vi "Write Measurement Values.vi"(0 "Selected Part Name":string="1891", 2 "RC JSON variant in":variant, 5 "Input Data Cluster":T1, 7 "Input File Paths Cluster":T5={"JSON Default filepath in"=path "F:/User Interface Testbench/Configuration file/Zengage System JSON UI.json", "JSON RackController\n(Override) filepath in"=path "F:/User Interface Testbench/Configuration file/Rack Controller Override JSON UI.json", "JSON AlgoParameters\n(Override) filepath in"=path "F:/User Interface Testbench/Configuration file/Algorithm Override JSON.json"}, 9 "Measurements Cluster":T4={"Measurement Values"=[["L", "AET", "16", "2", "10", "2", "10", "1", "0"], ["W", "AET", "2.5", "-10", "100", "-10", "100", "1", "0"], ["I1", "Length", "9.5", "-10", "100", "-10", "100", "1", "0"], ["U", "Coord", "2.3", "2", "20", "-10", "100", "1", "0"]], "Enabled Disable Array"=[]}, 11 "error in":errorcluster, 12 "User interface enqueuer":refnum<class "Message Enqueuer.lvclass">, 13 "Algo JSON variant in":variant) -> (4 "RC JSON variant out":variant, 6 "Algo JSON variant out":variant, 15 "error out":errorcluster)   [LabVIEW 2019, in "ZenGage v3.0 UI.lvclass"]
uses:
  ZenGage v3.0 UI.lvclass
  User Interface Messages/User Interface messages/Display Popup Msg/DisplayPopup_UI.lvclass
  Common/Controls/Pop-up Input.ctl
  <vilib>/ActorFramework/Message Enqueuer/Message Enqueuer.lvclass
  Type Definitions/Edit tolerance settings/Rack Selection.ctl
  <vilib>/Utility/miscctls.llb/LVPoint32TypeDef.ctl
  Type Definitions/Edit tolerance settings/Edit Tolerance Input.ctl
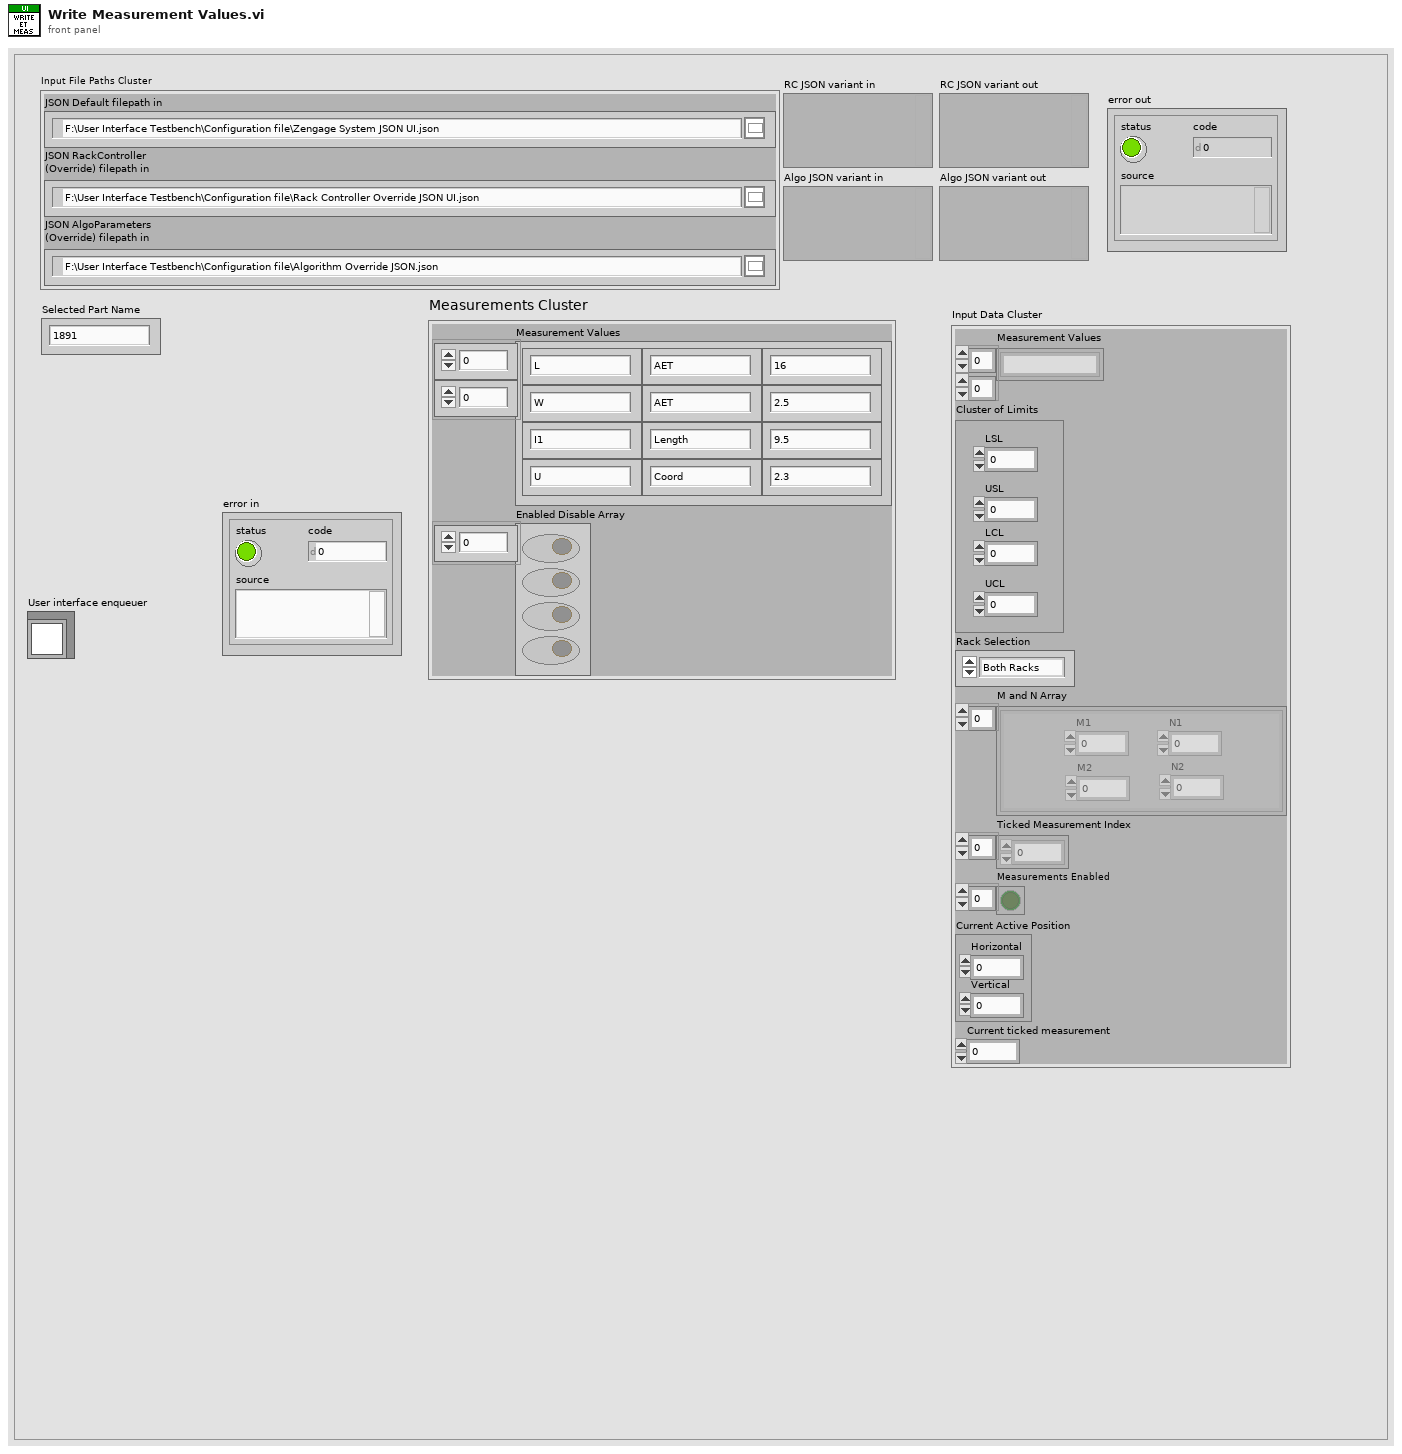
[diagram p1: front panel]
types:
  T1 = typedef "ZenGage v3.0 UI.lvclass/Edit Tolerance Input.ctl" = cluster{"Measurement Values":string[][], "Cluster of Limits":cluster{"LSL":dbl, "USL":dbl, "LCL":dbl, "UCL":dbl}, "Rack Selection":T2, "M and N Array":cluster{"M1":u64, "M2":u64, "N1":u64, "N2":u64}[], "Ticked Measurement Index":u32[], "Measurements Enabled":bool[], "Current Active Position":T3, "Current ticked measurement":dbl}
  T2 = typedef "ZenGage v3.0 UI.lvclass/Rack Selection.ctl" = enum16{"Both Racks", "Rack 2", "Rack 1"}
  T3 = typedef "LVPoint32TypeDef.ctl" = cluster{"Horizontal":i32, "Vertical":i32}
  T4 = cluster{"Measurement Values":string[][], "Enabled Disable Array":bool[]}
  T5 = cluster{"JSON Default filepath in":path, "JSON RackController\n(Override) filepath in":path, "JSON AlgoParameters\n(Override) filepath in":path}
  T6 = typedef "Pop-up Input.ctl" = cluster{"Pop-up Type":enum16{"Open Logo Display", "Close Logo Display", "Open Loading Bar", "Close Loading Bar", "Open Alert Display", "Close Alert Display", "One button dialog box", "Two button dialog box", "User Authentication"}, "Title":string, "Message":string, "Button 1 Text":string, "Button 2 Text":string, "Show Close? T/F":bool, "Title Blink? T/F":bool, "Title Blink Colour":u32}
  T7 = cluster{"Tolerance Limits":dbl[][], "Measurement Enable":bool[], "Bias Correction":dbl[], "Linearity Correction":dbl[], "Measurement names":string[]}
  T8 = cluster{"M1":u64, "M2":u64, "N1":u64, "N2":u64}[]
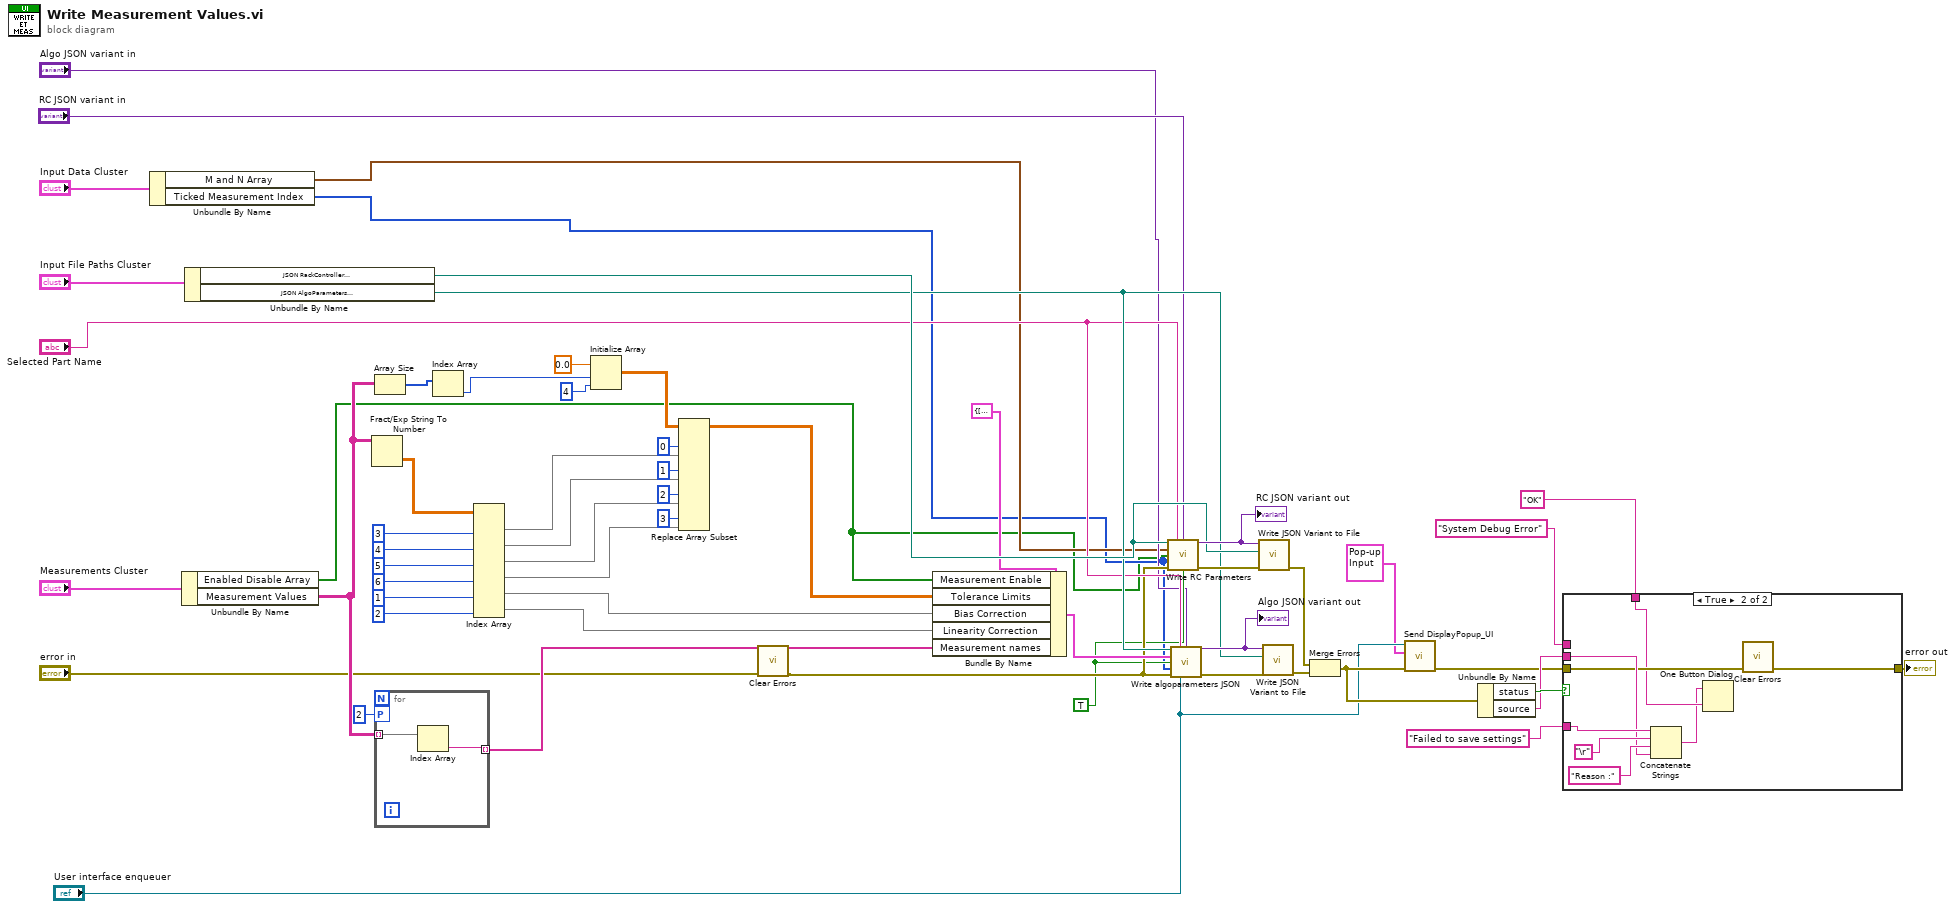
[diagram p0: block diagram]
diagram:
  w12 = TRUE
  n1 = Unbundle By Name("Input Data Cluster") -> ("M and N Array"=w5:T8, "Ticked Measurement Index"=w4:u32[])
  n2 = Unbundle By Name("Measurements Cluster") -> ("Enabled Disable Array"=w1:bool[], "Measurement Values"=w16:string[][])
  n3 = Unbundle By Name("Input File Paths Cluster") -> ("JSON RackController\n(Override) filepath in"=w44:path, "JSON AlgoParameters\n(Override) filepath in"=w43:path)
  n4 = Fract/Exp String To Number(string=w16) -> (number=w54:dbl[][])  [unwired: 3 in, 1 out]
  n5 = Array Size(array=w16) -> (size(s)=w31:i32[])
  n6 = for {
    tunnel: w16 -> [w60] mode=indexing
    tunnel: [w59] -> w15 mode=indexing
    workers-P: 2 -> [_]
    n7 = Index Array(array=w60) -> (element=w59:string)  [unwired: 1 in]
  }
  n8 = Index Array(array=w31) -> (element=w30:i32)  [unwired: 1 in]
  n9 = Index Array(array=w54, index (col) #1=3 ("index (row)"), index (col) #2=4 ("index (row)"), index (col) #3=5 ("index (row)"), index (col) #4=6 ("index (row)"), index (col) #5=1 ("index (row)"), index (col) #6=2 ("index (row)")) -> (element #1=w53:dbl[], element #2=w52:dbl[], element #3=w51:dbl[], element #4=w50:dbl[], element #5=w40:dbl[], element #6=w39:dbl[])  [unwired: 6 in]
  n10 = Initialize Array(0.0, w30, 4 ("dimension size")) -> (w55:dbl[][])
  n11 = Replace Array Subset(array=w55, new element #1=w53, index (col) #1=0 ("disabled index (col)"), new element #2=w52, index (col) #2=1 ("index (col)"), new element #3=w51, index (col) #3=2 ("index (col)"), new element #4=w50, index (col) #4=3 ("index (col)")) -> (w36:dbl[][])  [unwired: 4 in]
  n12 = call <vilib>:"Clear Errors.vi"("error in (no error)"="error in") -> ("error out"=w13:errorcluster)  [unwired: 5 in, 1 out]
  n13 = Bundle By Name(cluster=T7 {"Tolerance Limits"=[[3.9, 4.3, 3.9, 4.3], [15.2, 15.8, 15.2, 15.8], [15.2, 15.8, 15.2, 15.8], [15.2, 15.8, 15.2, 15.8], [15.2, 15.8, 15.2, 15.8], [15.2, 15.8, 15.2, 15.8], [15.2, 15.8, 15.2, 15.8]], "Measurement Enable"=[TRUE, TRUE, TRUE, TRUE, TRUE, TRUE, TRUE], "Bias Correction"=[-0.144, -0.779, -0.779, -0.779, -0.779, -0.779, -0.779], "Linearity Correction"=[1.0, 1.047, 1.047, 1.047, 1.047, 1.047, 1.047], "Measurement names"=[]} ("Input data cluster"), "Measurement Enable"=w1, "Tolerance Limits"=w36, "Bias Correction"=w40, "Linearity Correction"=w39, "Measurement names"=w15) -> (w17:T7)
  n14 = call "Write RC Parameters.vi"("JSON FilePath"=w44, "Part Name"="Selected Part Name", "RC parameters variant"="RC JSON variant in", "M and N array"=w5, "Enabled Disable Array"=w1, "Ticked measurements"=w4, "error in (no error)"=w13, "Variant"=w12) -> ("JSON Variant"=w45:variant, "error out"=w48:errorcluster)  [unwired: 6 in]
  "RC JSON variant out" <- w45
  n15 = call "Write algoparameters JSON.vi"("JSON FilePath"=w43, "Part Name"="Selected Part Name", "Algo override variant"="Algo JSON variant in", "Input data cluster"=w17, "Variant"=w12, "Ticked measurements"=w4, "error in (no error)"=w13, "User interface enqueuer"="User interface enqueuer") -> ("JSON Variant"=w46:variant, "error out"=w47:errorcluster)  [unwired: 6 in]
  "Algo JSON variant out" <- w46
  n16 = call <vilib>:"Write JSON Variant to File.vi"("Error In"=w48, "file (use dialog)"=w44, "JSON Varaint"=w45) -> ("error out"=w41:errorcluster)  [unwired: 8 in]
  n17 = call <vilib>:"Write JSON Variant to File.vi"("Error In"=w47, "file (use dialog)"=w43, "JSON Varaint"=w46) -> ("error out"=w42:errorcluster)  [unwired: 8 in]
  n18 = Merge Errors(w41, w42) -> (w9:errorcluster)
  n19 = call "Send DisplayPopup_UI.vi"("error in (no error)"=w9, "PopupDetails"=T6 {"Pop-up Type"=enum."Close Loading Bar", "Title"="", "Message"="", "Button 1 Text"="", "Button 2 Text"="", "Show Close? T/F"=FALSE, "Title Blink? T/F"=FALSE, "Title Blink Colour"=0}, "Message Enqueuer"="User interface enqueuer") -> ("error out"=w8:errorcluster)  [unwired: 7 in, 1 out]
  n20 = Unbundle By Name(w9) -> ("status"=w23:bool, "source"=w22:string)
  n21 = case shown="True" w23 {
    tunnel: "Failed to save settings" ("Message in") -> [_ w69]
    tunnel: w22 -> [_ w66]
    tunnel: w8 -> [w61 w64]
    tunnel: [w61 w65] -> w19
    tunnel: "System Debug Error" ("Dialogbox header") -> [_ _]
    tunnel: "OK" ("Button Name") -> [_ w63]
    frame False {
    }
    frame True {
      n22 = Concatenate Strings(w69, "\r", "Reason :" ("string"), w66) -> (w62:string)
      n23 = One Button Dialog(message=w62, button name ("OK")=w63) -> ()  [unwired: 1 out]
      n24 = call <vilib>:"Clear Errors.vi"("error in (no error)"=w64) -> ("error out"=w65:errorcluster)  [unwired: 5 in, 1 out]
    }
  }
  "error out" <- w19
